vi "APLUS Get Data.vi"(5 "Use String Data?":bool=TRUE, 7 "Debug":bool, 8 "error in (no error)":errorcluster, 10 "Reset WattHours":bool, 11 "Modbus Master in":refnum<class "Modbus Master.lvclass">) -> (0 "error out":errorcluster, 1 "APLUS Data":string[][](array[string]), 2 "PowerData":T2 {"Voltage (V):Element 1 Avg" format="%.3g"; "Voltage (V):Element 2 Avg" format="%.3g"; "Max Watt Hours" format="%.3g"; "Power Factor:Element 2" format="%.3g"; "Power Factor:Element 1" format="%.3g"; "Apparent Power (VA):Element 2" format="%.3g"; "Apparent Power (VA):Element 1" format="%.3g"; "Frequency (Hz):Element 1" format="%.3g"; "Time:Element 1" format="%.3g"; "Voltage Crest Factor:Element 2" format="%.3g"; "Voltage Crest Factor:Element 1" format="%.3g"; "Voltage Harmonic (%):Element 2" format="%.3g"; "Voltage Harmonic (%):Element 1" format="%.3g"; "Current Crest Factor:Element 2" format="%.3g"; "Current Crest Factor:Element 1" format="%.3g"; "Voltage (V):Element 1" format="%.3g"; "Voltage (V):Element 2" format="%.3g"; "Watt Hours (Wh):Sigma" format="%.3f"; "Power (W):Sigma" format="%.3g"; "Current (A):Element 2" format="%.3e"; "Current (A):Element 1" format="%.3e"}, 3 "Modbus Master out":refnum<class "Modbus Master.lvclass">, 4 "Power":sgl, 6 "APLUS DBL Data":dbl[](array[numeric]))   [LabVIEW 2020]
uses:
  <vilib>/NI/Modbus Library/API/Master/Modbus Master.lvclass
  Trunk/Utility/Type Definitions/UTILITY Power Data.ctl
  Type Definitions/APLUS Commands.ctl
panel:
  in  "System Type":T1=2199 items=["L1 Voltage (V) -14"=99, "L1 Voltage (V) -4U"=101, "L2 Voltage (V) -4U"=103, "L1 RMS Current (Amps) -14"=115, "L1 RMS Current (Amps) -4U"=117, "L2 RMS Current (Amps) -4U"=119, "Frequency (Hz) -All"=157, "Sys Power (Watts)-14"=133, "L1 Power (Watts)-4U"=135, "L2 Power (Watts)-4U"=137, "L1 Power Factor-14"=159, "L1 Power Factor-4U"=161, "L2 Power Factor-4U"=163, "L1 Apparent Power (VA)-14"=149, "L1 Apparent Power (VA)-4U"=151, "L2 Apparent Power (VA)-4U"=153, "Voltage Total Harmonic Distortion (%)-All"=235, "Active Energy Incoming-14"=1579, "Unit Factor-14"=1627, "Remainder Active Energy Incoming-14"=5999, "System Type"=2199]
  out "Holding Registers":u16[](array[numeric])
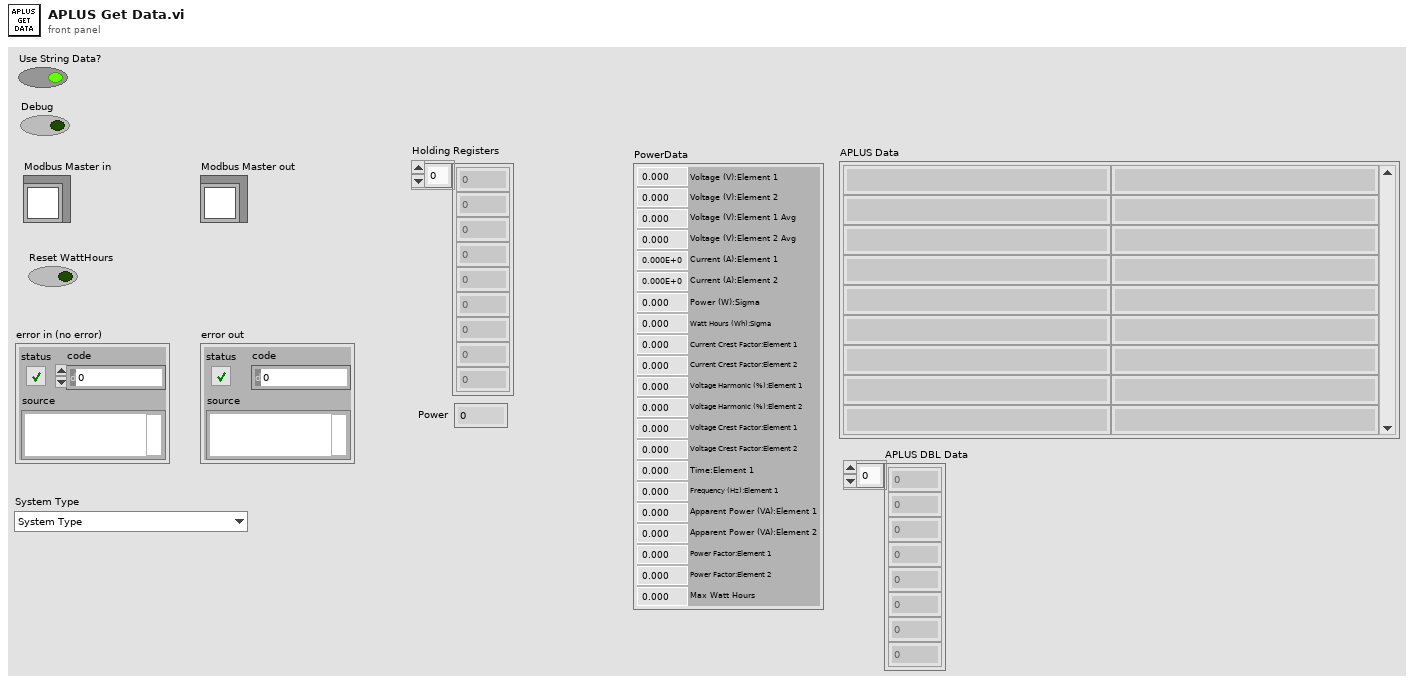
[diagram p1: front panel]
types:
  T1 = typedef "APLUS Commands.ctl" = u16
  T2 = typedef "UTILITY Power Data.ctl" = cluster{"Current (A):Element 1":dbl, "Current (A):Element 2":dbl, "Power (W):Sigma":dbl, "Watt Hours (Wh):Sigma":dbl, "Voltage (V):Element 2":dbl, "Voltage (V):Element 1":dbl, "Current Crest Factor:Element 1":dbl, "Current Crest Factor:Element 2":dbl, "Voltage Harmonic (%):Element 1":dbl, "Voltage Harmonic (%):Element 2":dbl, "Voltage Crest Factor:Element 1":dbl, "Voltage Crest Factor:Element 2":dbl, "Time:Element 1":dbl, "Frequency (Hz):Element 1":dbl, "Apparent Power (VA):Element 1":dbl, "Apparent Power (VA):Element 2":dbl, "Power Factor:Element 1":dbl, "Power Factor:Element 2":dbl, "Max Watt Hours":dbl, "Voltage (V):Element 2 Avg":dbl, "Voltage (V):Element 1 Avg":dbl}
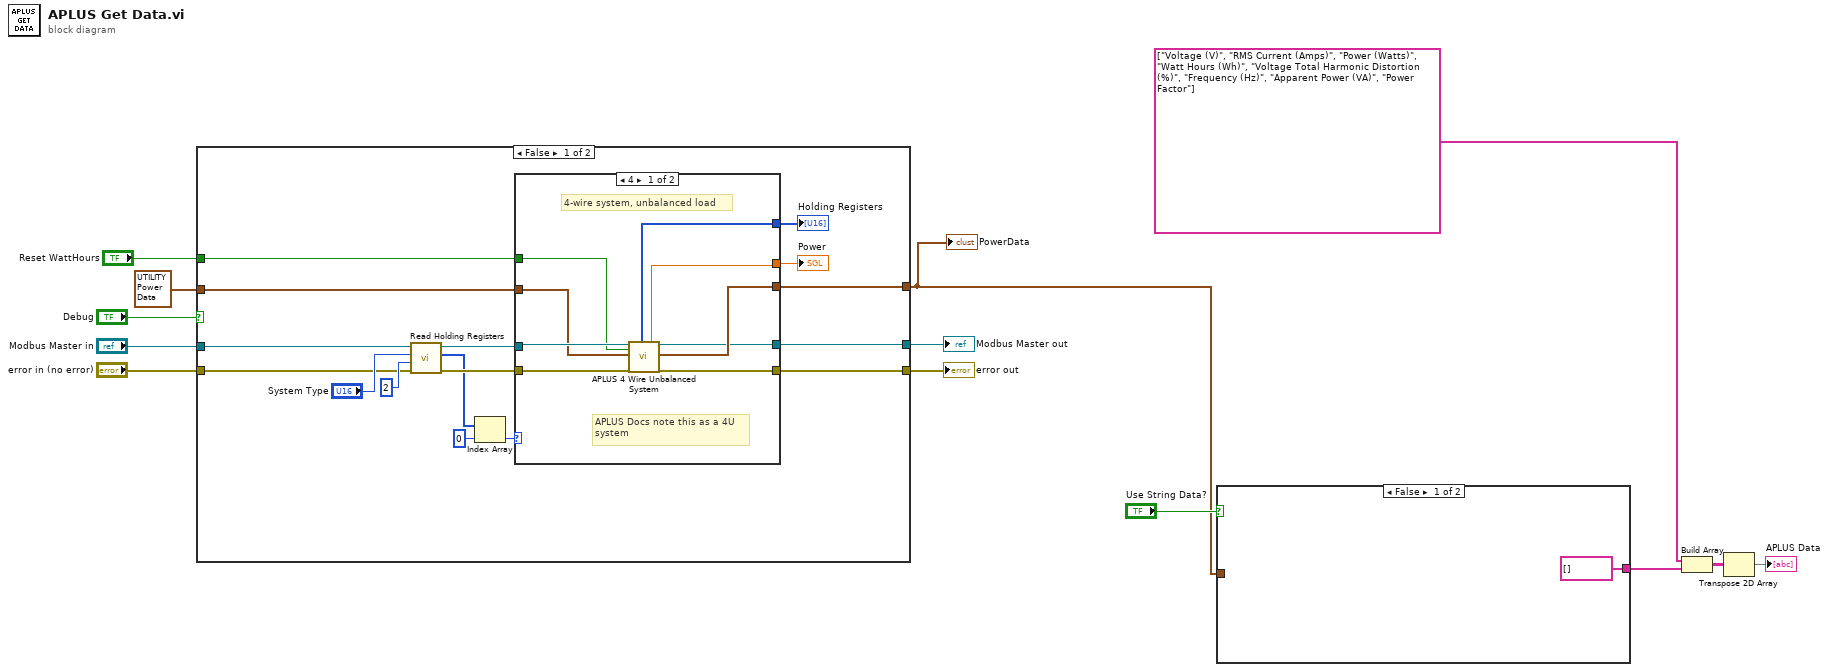
[diagram p0: block diagram]
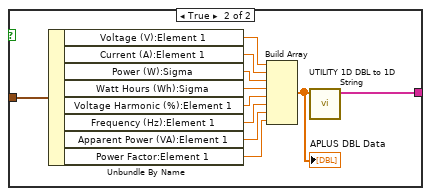
[diagram p2: hidden frame]
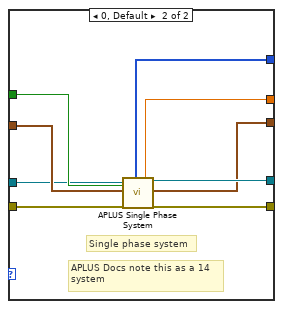
[diagram p3: hidden frame]
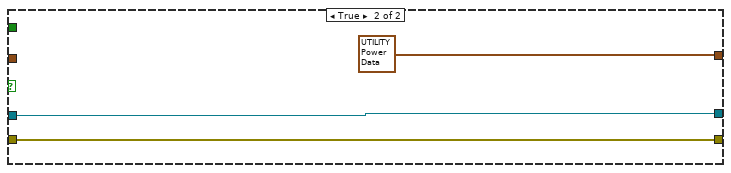
[diagram p4: hidden frame]
diagram:
  n1 = case shown="False" "Debug" {
    tunnel: "Modbus Master in" -> [w22 w49]
    tunnel: "error in (no error)" -> [w21 w50]
    tunnel: [w29 w50] -> w11
    tunnel: [w28 w49] -> w10
    tunnel: "Reset WattHours" -> [w27 _]
    tunnel: [w26 T2 {"Current (A):Element 1"=0.0, "Current (A):Element 2"=0.0, "Power (W):Sigma"=0.0, "Watt Hours (Wh):Sigma"=0.0, "Voltage (V):Element 2"=0.0, "Voltage (V):Element 1"=0.0, "Current Crest Factor:Element 1"=0.0, "Current Crest Factor:Element 2"=0.0, "Voltage Harmonic (%):Element 1"=0.0, "Voltage Harmonic (%):Element 2"=0.0, "Voltage Crest Factor:Element 1"=0.0, "Voltage Crest Factor:Element 2"=0.0, "Time:Element 1"=0.0, "Frequency (Hz):Element 1"=0.0, "Apparent Power (VA):Element 1"=0.0, "Apparent Power (VA):Element 2"=0.0, "Power Factor:Element 1"=0.0, "Power Factor:Element 2"=0.0, "Max Watt Hours"=0.0, "Voltage (V):Element 2 Avg"=0.0, "Voltage (V):Element 1 Avg"=0.0} ("PowerData")] -> w1
    tunnel: T2 {"Current (A):Element 1"=236.2, "Current (A):Element 2"=17.749, "Power (W):Sigma"=4192.0, "Watt Hours (Wh):Sigma"=0.0, "Voltage (V):Element 2"=236.2, "Voltage (V):Element 1"=236.2, "Current Crest Factor:Element 1"=0.0, "Current Crest Factor:Element 2"=0.0, "Voltage Harmonic (%):Element 1"=0.0, "Voltage Harmonic (%):Element 2"=0.0, "Voltage Crest Factor:Element 1"=0.0, "Voltage Crest Factor:Element 2"=0.0, "Time:Element 1"=0.0, "Frequency (Hz):Element 1"=0.0, "Apparent Power (VA):Element 1"=0.0, "Apparent Power (VA):Element 2"=0.0, "Power Factor:Element 1"=0.0, "Power Factor:Element 2"=0.0, "Max Watt Hours"=0.0, "Voltage (V):Element 2 Avg"=0.0, "Voltage (V):Element 1 Avg"=0.0} ("PowerData") -> [w25 _]
    frame False {
      n2 = call-dynamic "Read Holding Registers.vi"("error in"=w21, "number of inputs"=u16 2 ("Quantity"), "starting address"="System Type", "Modbus master in"=w22) -> ("error out"=w19:errorcluster, "register values"=w18:u16[], "Modbus master out"=w20:refnum<class "Modbus Master.lvclass">)  [unwired: 5 in]
      n3 = Index Array(array=w18, index=0) -> (element=w16:u16)
      n4 = case shown="4" w16 {
        tunnel: [w37 w47] -> w29
        tunnel: [w35 w46] -> w28
        tunnel: w27 -> [w33 w45]
        tunnel: [w36 w44] -> w26
        tunnel: w25 -> [w32 w43]
        tunnel: w20 -> [w34 w42]
        tunnel: w19 -> [w38 w41]
        tunnel: [w30 w40] -> w15
        tunnel: [w31 w39] -> w14
        frame 4 {
          # "APLUS Docs note this as a 4U\nsystem"
          # "4-wire system, unbalanced load"
          n5 = call "APLUS 4 Wire Unbalanced System.vi"("Modbus Master in"=w34, "Reset WattHours"=w33, "Power Input"=w32, "error in (no error)"=w38) -> ("Holding Registers"=w30:u16[], "Power"=w31:sgl, "Modbus Master out"=w35:refnum<class "Modbus Master.lvclass">, "PowerData"=w36:T2, "error out"=w37:errorcluster)  [unwired: 11 in]
        }
        frame 0, Default {
          # "APLUS Docs note this as a 14\nsystem"
          # "Single phase system"
          n6 = call "APLUS Single Phase System.vi"("Modbus Master in"=w42, "Reset WattHours"=w45, "Power Input"=w43, "error in (no error)"=w41) -> ("Holding Registers"=w40:u16[], "Power"=w39:sgl, "Modbus Master out"=w46:refnum<class "Modbus Master.lvclass">, "PowerData"=w44:T2, "error out"=w47:errorcluster)  [unwired: 11 in]
        }
      }
      "Holding Registers" <- w15
      "Power" <- w14
    }
    frame True {
    }
  }
  "error out" <- w11
  "Modbus Master out" <- w10
  "PowerData" <- w1
  n7 = case shown="False" "Use String Data?" {
    tunnel: w1 -> [_ w53]
    tunnel: [string[] [] ("1D String") w52] -> w4
    frame False {
    }
    frame True {
      n8 = Unbundle By Name(w53) -> ("Voltage (V):Element 1"=w61:dbl, "Current (A):Element 1"=w60:dbl, "Power (W):Sigma"=w59:dbl, "Watt Hours (Wh):Sigma"=w58:dbl, "Voltage Harmonic (%):Element 1"=w57:dbl, "Frequency (Hz):Element 1"=w56:dbl, "Apparent Power (VA):Element 1"=w55:dbl, "Power Factor:Element 1"=w54:dbl)
      n9 = Build Array(w61, w60, w59, w58, w57, w56, w55, w54) -> (w62:dbl[])
      "APLUS DBL Data" <- w62
      n10 = call "UTILITY 1D DBL to 1D String.vi"("1D DBL"=w62) -> ("1D String"=w52:string[])  [unwired: 10 in]
    }
  }
  n11 = Build Array(string[] ["Voltage (V)", "RMS Current (Amps)", "Power (Watts)", "Watt Hours (Wh)", "Voltage Total Harmonic Distortion (%)", "Frequency (Hz)", "Apparent Power (VA)", "Power Factor"], w4) -> (w6:string[][])
  n12 = Transpose 2D Array(2D array=w6) -> (transposed array=→"APLUS Data":string[][])
